vi "subSaveAsBin_NW348.vi"(5 "Delete .dcimg?":bool, 7 "Save Text file?":bool, 8 "Error in":errorcluster, 10 "Text":string, 11 ".dcimg file name":path) -> (0 "Error out":errorcluster, 4 "text path":path)   [LabVIEW 2013]
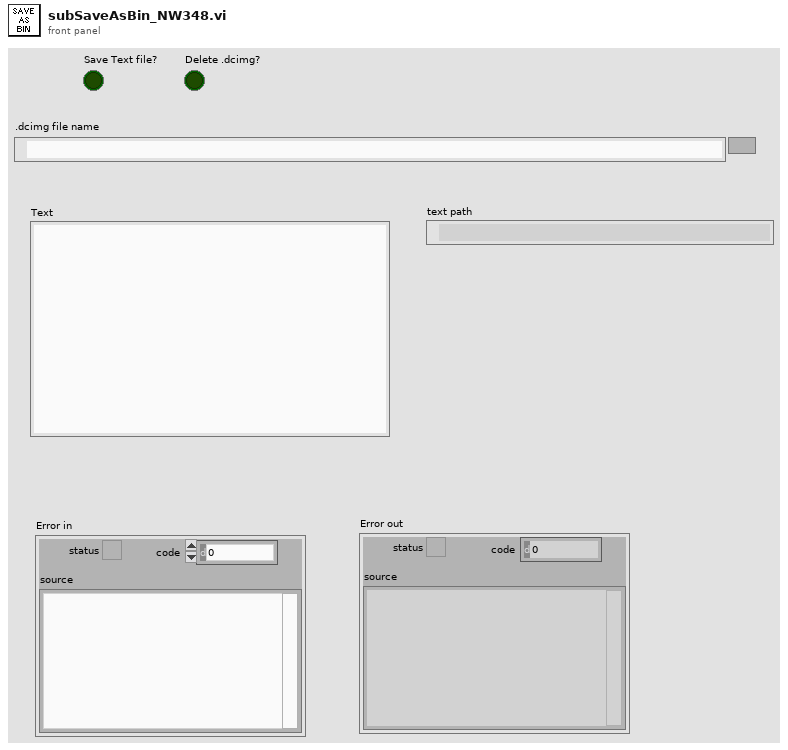
[diagram p1: front panel]
types:
  T1 = enum16{"open", "replace", "create", "open or create", "replace or create", "replace or create with confirmation"}
  T2 = enum16{"big-endian, network order", "native, host order", "little-endian"}
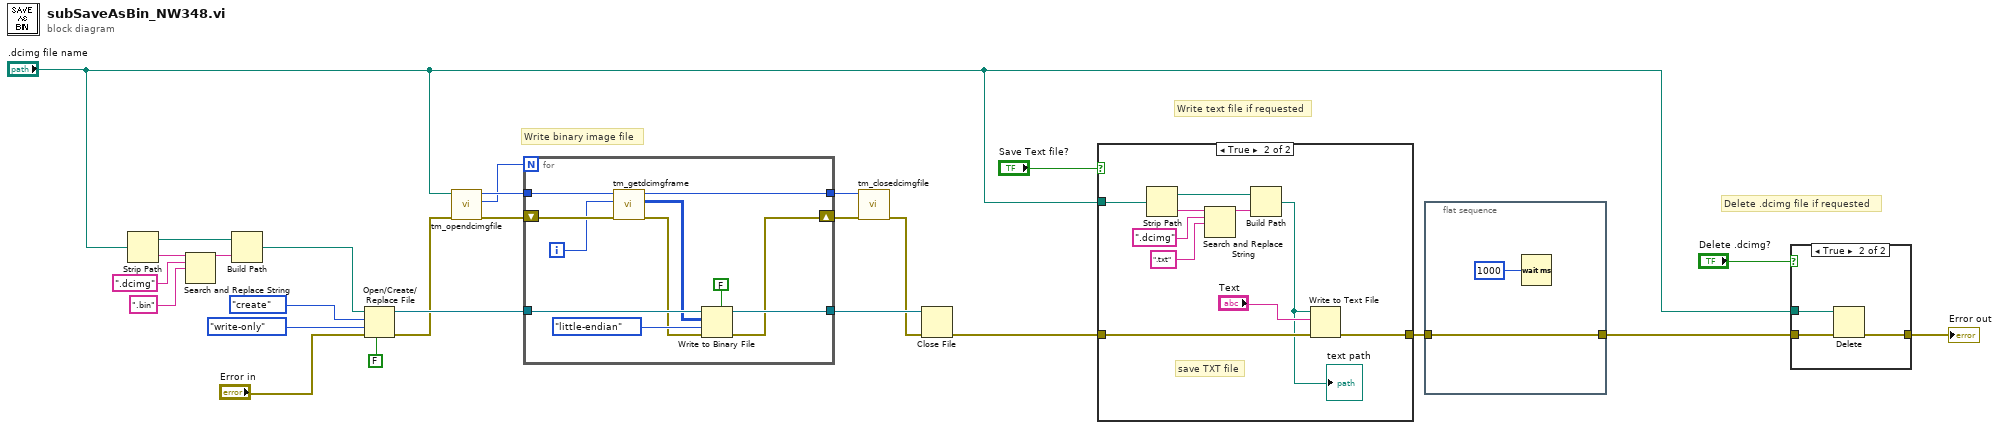
[diagram p0: block diagram]
diagram:
  # "Delete .dcimg file if requested"
  # "Write binary image file"
  # "Write text file if requested"
  n1 = Strip Path(path=".dcimg file name") -> (stripped path=w16:path, name=w13:string)
  n2 = Search and Replace String(input string=w13, search string=".dcimg", replace string=".bin" ("replace string (\"\")")) -> (result string=w17:string)  [unwired: 5 in, 3 out]
  n3 = Build Path(base path=w16, name or relative path=w17) -> (appended path=w12:path)
  n4 = Open/Create/Replace File(file path (use dialog)=w12, error in="Error in", operation (0:open)=T1."create", access (0:read/write)=enum16{"read/write", "read-only", "write-only"}."write-only", disable buffering (F)=FALSE) -> (refnum out=w26:refnum<file>, error out=w9:errorcluster)  [unwired: 1 in, 1 out]
  n5 = call <userlib>:"tm_opendcimgfile.vi"("error in (no error)"=w9, "Path"=".dcimg file name") -> ("error out"=w24:errorcluster, "Total Frames"=w7:i32, "File Handle"=w25:u32)  [unwired: 7 in]
  n6 = for {
    N: w7 -> [_]
    shift-right: [w28] -> w23
    shift-left: w24 -> [w37]
    tunnel: w25 -> [w36]
    tunnel: [w35] -> w22
    tunnel: w26 -> [w33]
    tunnel: [w30] -> w21
    i -> [w29]
    n7 = call <userlib>:"tm_getdcimgframe.vi"("error in (no error)"=w37, "Frame Index"=w29, "File Handle in"=w36) -> ("error out"=w27:errorcluster, "Data"=w31:u16[][], "File Handle out"=w35:u32)  [unwired: 5 in, 1 out]
    n8 = Write to Binary File(file (use dialog)=w33, data=w31, error in=w27, 5:FALSE, 9:T2."little-endian" ("byte order (0:big-endian, network order)")) -> (refnum out=w30:refnum<file>, error out=w28:errorcluster)  [unwired: 1 in, 1 out]
  }
  n9 = call <userlib>:"tm_closedcimgfile.vi"("error in (no error)"=w23, "File Handle"=w22) -> ("error out"=w8:errorcluster)  [unwired: 9 in]
  n10 = Close File(refnum=w21, error in=w8) -> (error out=w3:errorcluster)  [unwired: 1 out]
  n11 = case shown="True" "Save Text file?" {
    tunnel: ".dcimg file name" -> [_ w43]
    tunnel: w3 -> [w38 w42]
    tunnel: [w38 w41] -> w2
    frame False {
    }
    frame True {
      # "save TXT file"
      n12 = Strip Path(path=w43) -> (stripped path=w47:path, name=w44:string)
      n13 = Search and Replace String(input string=w44, search string=".dcimg", replace string=".txt" ("replace string (\"\")")) -> (result string=w48:string)  [unwired: 5 in, 3 out]
      n14 = Build Path(base path=w47, name or relative path=w48) -> (appended path=w39:path)
      "text path" <- w39
      n15 = Write to Text File(file (use dialog)=w39, text="Text", error in=w42) -> (error out=w41:errorcluster)  [unwired: 1 in, 2 out]
    }
  }
  n16 = flat-sequence {
    tunnel: w2 -> [w50]
    tunnel: [w50] -> w4
    frame #0 {
      n17 = Wait (ms)(milliseconds to wait=u32 1000) -> ()  [unwired: 1 out]
    }
  }
  n18 = case shown="True" "Delete .dcimg?" {
    tunnel: w4 -> [w51 w54]
    tunnel: [w51 w53] -> w6
    tunnel: ".dcimg file name" -> [_ w52]
    frame False {
    }
    frame True {
      n19 = Delete(path (use dialog)=w52, error in=w54) -> (error out=w53:errorcluster)  [unwired: 3 in, 2 out]
    }
  }
  "Error out" <- w6
